vi "SeverityString.vi"(8 "error in (no error)":errorcluster, 11 "Severity":T1=enum."INFO") -> (0 "error out":errorcluster, 3 "SeverityString":string)   [LabVIEW 2026, in "Lumberjack.lvlib"]
doc: "Converts a Severity enum to its member-name string (OFF, FATAL, ERROR, WARN, INFO, DEBUG, TRACE, ALL).\nDoubles as the level token in log output; round-trip partner of SeverityFromString. Pure; no state, no I/O.\nLumberjack.lvlib, community (friend of Tests.lvlib)."
uses:
  Lumberjack.lvlib
  TypeDefs/Severity.ctl
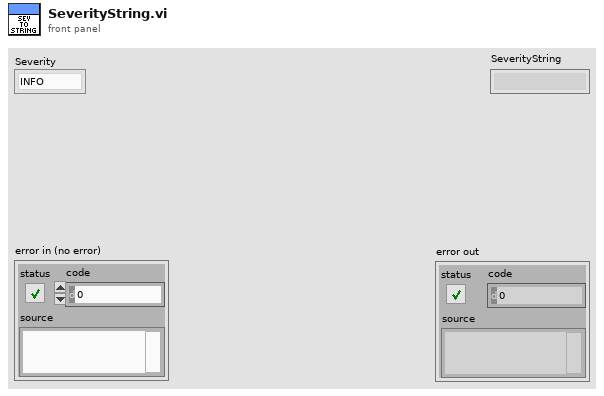
[diagram p1: front panel]
types:
  T1 = typedef "Lumberjack.lvlib/Severity.ctl" = enum16{"OFF", "FATAL", "ERROR", "WARN", "INFO", "DEBUG", "TRACE", "ALL"}
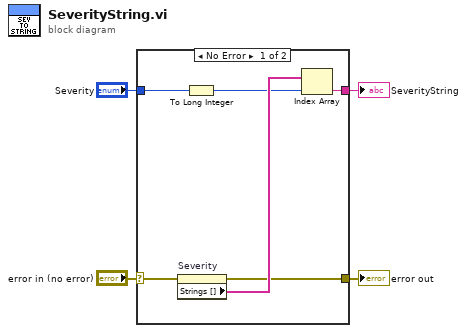
[diagram p0: block diagram]
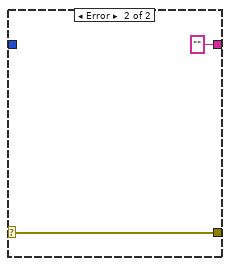
[diagram p2: hidden frame]
diagram:
  n1 = case shown="No Error" "error in (no error)" {
    selector: "error in (no error)" -> [w5 w12]
    tunnel: [w8 ""] -> w1
    tunnel: [w7 w12] -> w2
    tunnel: "Severity" -> [w6 _]
    frame No Error {
      n2 = property on="Severity" class="Enum (strict)"(error in=w5) -> (error out=w7:errorcluster, "Strings []"=w10:string[])  [unwired: 1 in, 1 out]
      n3 = To Long Integer(number=w6) -> (32bit integer=w9:i32)
      n4 = Index Array(array=w10, index=w9) -> (element=w8:string)
    }
    frame Error {
    }
  }
  "error out" <- w2
  "SeverityString" <- w1
